vi "Get Actual Temperature.vi"(8 "error in (no error)":errorcluster, 10 "Time Stamp":timestamp, 11 "Thermal Chamber Response Simlator In":refnum<class "Thermal Chamber Response Simlator.lvclass">) -> (0 "error out":errorcluster, 2 "Actual Temperature [degC]":dbl, 3 "Thermal Chamber Response Simlator Out":refnum<class "Thermal Chamber Response Simlator.lvclass">)   [LabVIEW 2020, in "Thermal Chamber Response Simlator.lvclass"]
uses:
  Thermal Chamber Response Simlator.lvclass
  Thermal Chamber Response Simlator.lvclass/Thermal Chamber Response Simlator.ctl
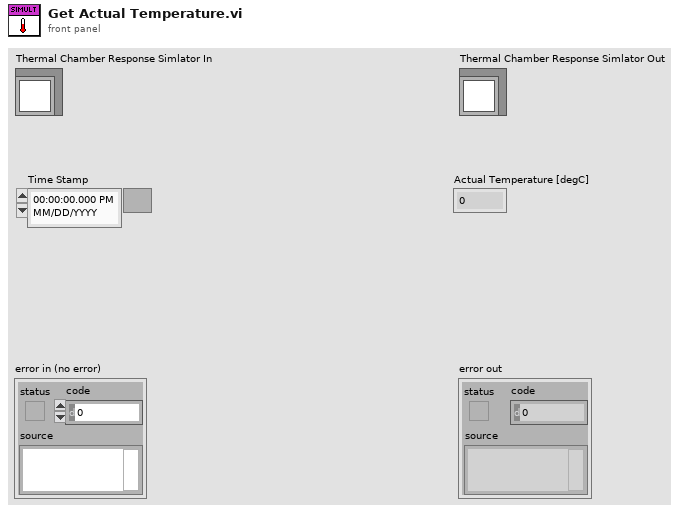
[diagram p1: front panel]
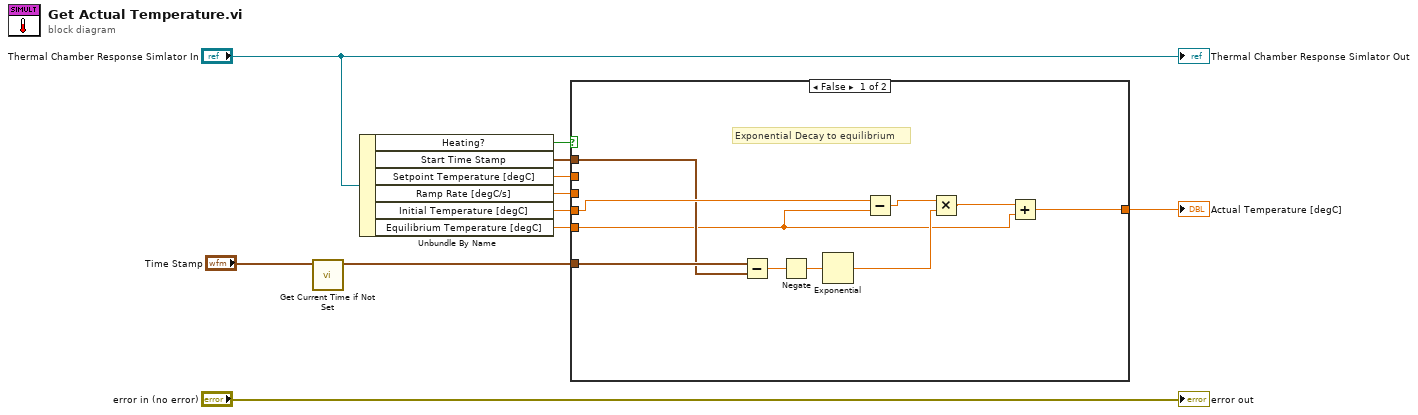
[diagram p0: block diagram]
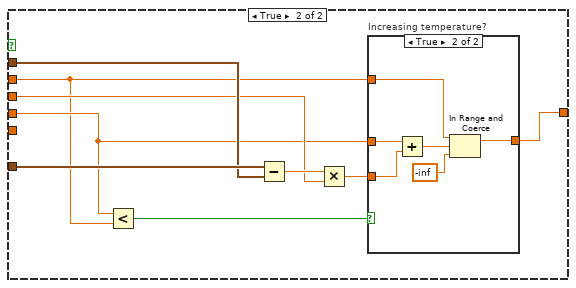
[diagram p2: hidden frame]
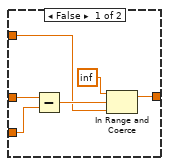
[diagram p3: hidden frame]
diagram:
  n1 = call "Get Current Time if Not Set.vi"("Start Time"="Time Stamp") -> ("seconds since 1Jan1904"=w8:timestamp)  [unwired: 10 in]
  n2 = Unbundle By Name("Thermal Chamber Response Simlator In") -> ("Heating?"=w2:bool, "Start Time Stamp"=w7:timestamp, "Setpoint Temperature [degC]"=w4:dbl, "Ramp Rate [degC/s]"=w6:dbl, "Initial Temperature [degC]"=w5:dbl, "Equilibrium Temperature [degC]"=w1:dbl)
  n3 = case shown="False" w2 {
    tunnel: w8 -> [w21 w30]
    tunnel: w7 -> [w15 w29]
    tunnel: w6 -> [_ w27]
    tunnel: w5 -> [w19 w25]
    tunnel: w4 -> [_ w23]
    tunnel: [w20 w22] -> w3
    tunnel: w1 -> [w12 _]
    frame False {
      # "Exponential Decay to equilibrium"
      n4 = Subtract(x=w21, y=w15) -> (x-y=w17:dbl)
      n5 = Negate(x=w17) -> (-x=w14:dbl)
      n6 = Exponential(1:w14) -> (0:w16:dbl)
      n7 = Subtract(x=w19, y=w12) -> (x-y=w13:dbl)
      n8 = Multiply(x=w13, y=w16) -> (x*y=w18:dbl)
      n9 = Add(x=w18, y=w12) -> (x+y=w20:dbl)
    }
    frame True {
      n10 = Less?(x=w25, y=w23) -> (x < y?=w24:bool)
      n11 = Subtract(x=w30, y=w29) -> (x-y=w28:dbl)
      n12 = Multiply(x=w28, y=w27) -> (x*y=w26:dbl)
      n13 = case "Increasing temperature?" shown="True" w24 {
        tunnel: w26 -> [w35 w42]
        tunnel: w25 -> [w36 w41]
        tunnel: w23 -> [w33 w38]
        tunnel: [w31 w37] -> w22
        frame False {
          n14 = Subtract(x=w36, y=w35) -> (x-y=w34:dbl)
          n15 = In Range and Coerce(upper limit=inf, x=w34, lower limit=w33) -> (coerced(x)=w31:dbl)  [unwired: 1 out]
        }
        frame True {
          n16 = Add(x=w41, y=w42) -> (x+y=w39:dbl)
          n17 = In Range and Coerce(upper limit=w38, x=w39, lower limit=-inf ("upper limit")) -> (coerced(x)=w37:dbl)  [unwired: 1 out]
        }
      }
    }
  }
  "Actual Temperature [degC]" <- w3
  "error out" <- "error in (no error)"
  "Thermal Chamber Response Simlator Out" <- "Thermal Chamber Response Simlator In"
